vi "OpenCurrentSource.vi"() -> (2 "error out":errorcluster, 3 "reference out":refnum<visa-resource-name>)   [LabVIEW 2009]
uses:
  <vilib>/Instr/_visa.llb/VISA Configure Serial Port (Instr).vi
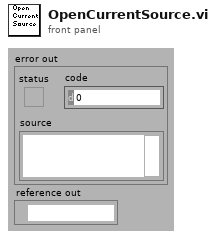
[diagram p1: front panel]
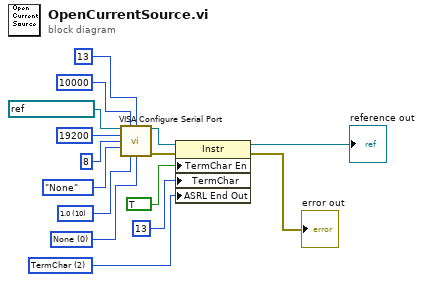
[diagram p0: block diagram]
diagram:
  w3 = u16 2 items=["None", "Last Bit", "TermChar", "Break"] ("Serial Settings:End Mode for Writes")
  w9 = u16 0 items=["None", "XON/XOFF", "RTS/CTS", "XON/XOFF & RTS/CTS", "DTR/DSR", "XON/XOFF & DTR/DSR"] ("flow control (0:none)")
  w10 = u16 10 items=["1.0"=10, "1.5"=15, "2.0"=20] ("stop bits (10: 1 bit)")
  n1 = call-poly "VISA Configure Serial Port"("VISA resource name"=refnum<visa-resource-name> "COM4", "timeout (10sec)"=u32 10000, "termination char\n(0xA = '\\n' = LF)"=u8 13 ("termination char\n(0xA = '\\n' = LF)"), "baud rate (9600)"=u32 19200, "data bits (8)"=u16 8, "parity (0:none)"=enum16{"None", "Odd", "Even", "Mark", "Space"}."None", "stop bits (10: 1 bit)"=w10, "flow control (0:none)"=w9) -> ("VISA resource name out"=w15:refnum<visa-resource-name>, "error out"=w8:errorcluster)  [unwired: 6 in]
  n2 = property class="Instr"(reference=w15, error in=w8, "TermChar En"=TRUE ("Message Based Settings:Termination Character Enable"), "TermChar"=u8 13 ("Message Based Settings:Termination Character"), "ASRL End Out"=w3) -> (reference out=→"reference out":refnum<visa-resource-name>, error out=→"error out":errorcluster)
